vi "MeasurementServer_Stop.vi"(0 "Server Information":T2, 1 "Event Registration Refnum":refnum<event-registration>, 3 "error in (no error)":errorcluster) -> (10 "error out":errorcluster)   [LabVIEW 2019, in "labview-grpc-measurement-server.lvlib"]
uses:
  labview-grpc-measurement-server.lvlib
  MeasurementServer_InvokeEventData.ctl
  MeasurementServer_gRPCid.ctl
  home/lvuser/ocv_labview_measurement_server.so
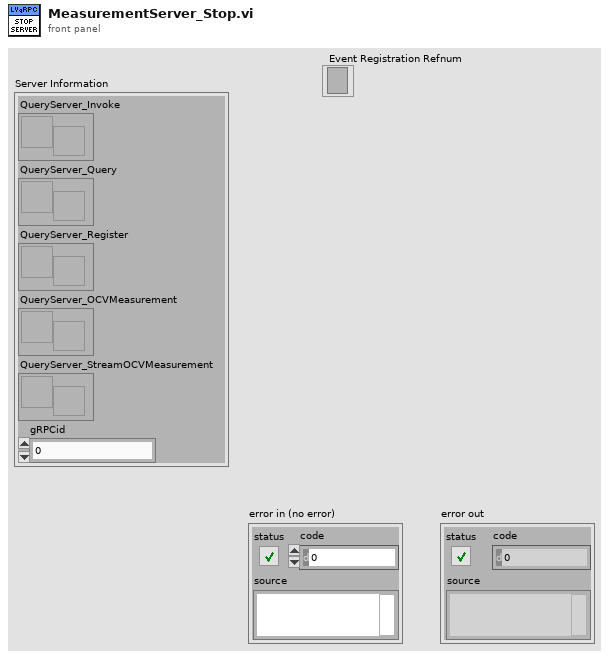
[diagram p1: front panel]
types:
  T1 = typedef "labview-grpc-measurement-server.lvlib/MeasurementServer_gRPCid.ctl" = u64
  T2 = cluster{"QueryServer_Invoke":refnum<user-event>, "QueryServer_Query":refnum<user-event>, "QueryServer_Register":refnum<user-event>, "QueryServer_OCVMeasurement":refnum<user-event>, "QueryServer_StreamOCVMeasurement":refnum<user-event>, "gRPCid":T1}
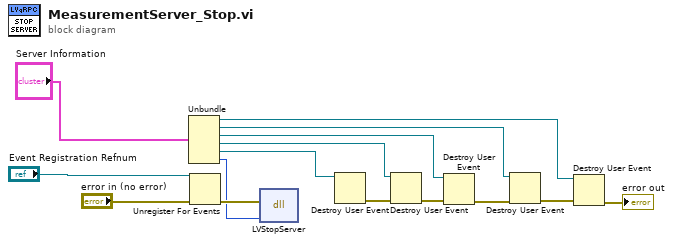
[diagram p0: block diagram]
diagram:
  n1 = Unbundle("Server Information") -> ("QueryServer_Invoke"=w8:refnum<user-event>, "QueryServer_Query"=w9:refnum<user-event>, "QueryServer_Register"=w10:refnum<user-event>, "QueryServer_OCVMeasurement"=w6:refnum<user-event>, "QueryServer_StreamOCVMeasurement"=w4:refnum<user-event>, "gRPCid"=w3:T1)
  n2 = Unregister For Events(event registration refnum="Event Registration Refnum", error in="error in (no error)") -> (error out=w15:errorcluster)
  n3 = dll-call lib="home/lvuser/ocv_labview_measurement_server.so" fn="LVStopServer"(error in=w15, "server"=w3) -> ()  [unwired: 4 in, 2 out]
  n4 = Destroy User Event(user event=w4) -> (error out=w5:errorcluster)  [unwired: 1 in]
  n5 = Destroy User Event(user event=w6, error in=w5) -> (error out=w7:errorcluster)
  n6 = Destroy User Event(user event=w10, error in=w7) -> (error out=w13:errorcluster)
  n7 = Destroy User Event(user event=w9, error in=w13) -> (error out=w12:errorcluster)
  n8 = Destroy User Event(user event=w8, error in=w12) -> (error out=→"error out":errorcluster)
